vi "setTics.vi"(6 "AdditionalTics":dbl[](array[numeric]), 7 "tics":T3={"ticMin"=0.0, "ticStep"=0.0, "ticMax"=0.0, "minorDivsPerMajor"=2, "ticSpacing"=enum."Auto Tics", "ticPosition"=enum."Inside, no mirror"}, 8 "AxisSpan":dbl, 9 "Axis":T2, 11 "String in":string) -> (0 "polarGrid":dbl, 3 "String out":string)   [LabVIEW 2013]
uses:
  tics.ctl
  axisName.ctl
  commandArray.ctl
panel:
  out "Commands":T1
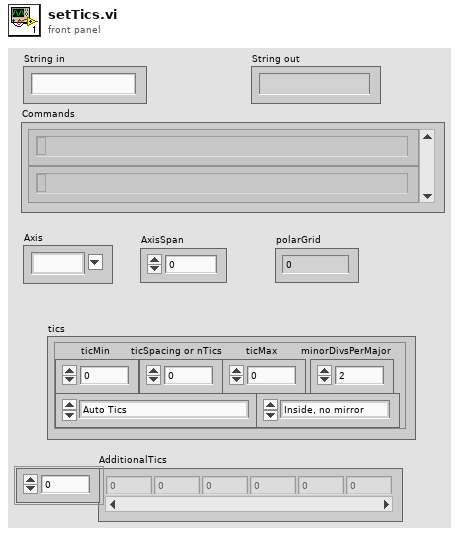
[diagram p1: front panel]
types:
  T1 = typedef "commandArray.ctl" = string[]
  T2 = typedef "axisName.ctl" = string
  T3 = typedef "tics.ctl" = cluster{"ticMin":dbl, "ticStep":dbl, "ticMax":dbl, "minorDivsPerMajor":i32, "ticSpacing":enum16{"Auto Tics", "Fixed spacing", "Fixed Minimum and Spacing", "Start, Spacing and Maximum", "Approx n Tics (rounded)"}, "ticPosition":enum16{"Inside, no mirror", "Inside, mirrored", "Outside, no mirror", "Outside, mirrored", "Invisible"}}
  T4 = enum16{"Auto Tics", "Fixed spacing", "Fixed Minimum and Spacing", "Start, Spacing and Maximum", "Approx n Tics (rounded)"}
  T5 = enum16{"Inside, no mirror", "Inside, mirrored", "Outside, no mirror", "Outside, mirrored", "Invisible"}
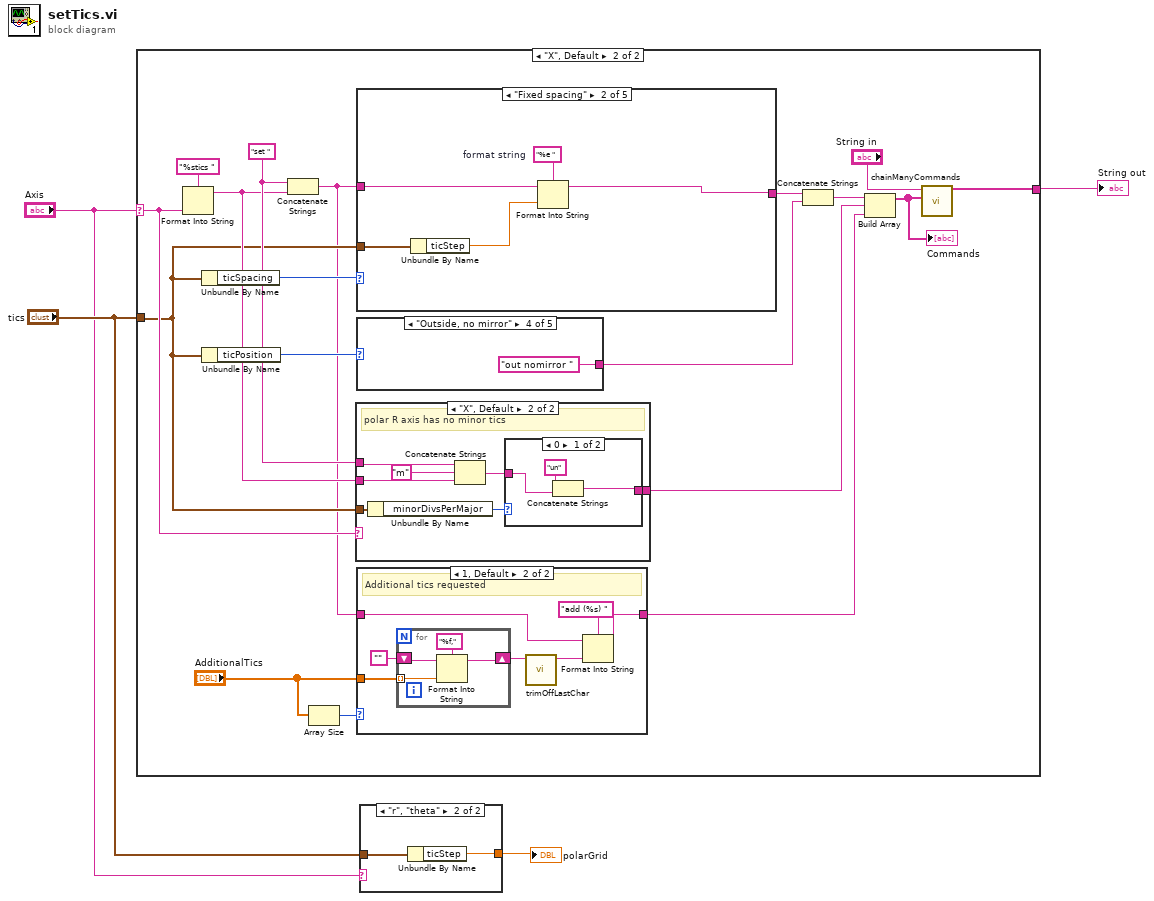
[diagram p0: block diagram]
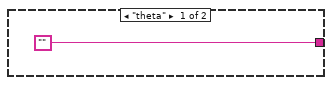
[diagram p2: hidden frame]
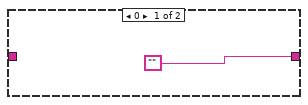
[diagram p3: hidden frame]
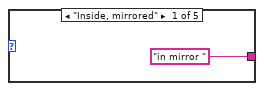
[diagram p4: hidden frame]
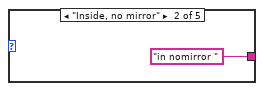
[diagram p5: hidden frame]
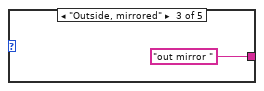
[diagram p6: hidden frame]
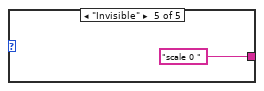
[diagram p7: hidden frame]
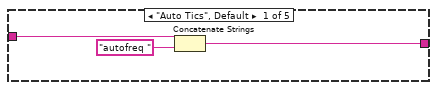
[diagram p8: hidden frame]
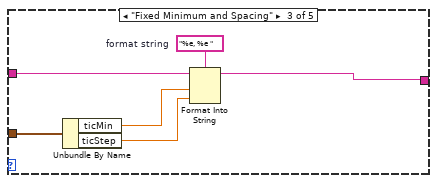
[diagram p9: hidden frame]
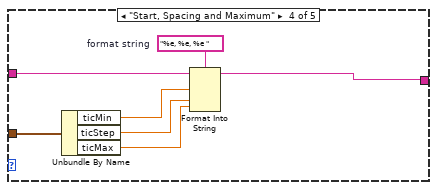
[diagram p10: hidden frame]
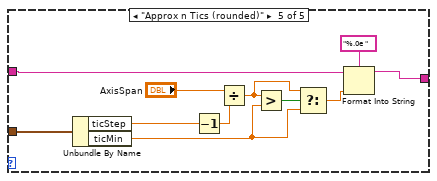
[diagram p11: hidden frame]
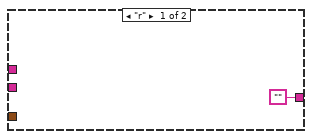
[diagram p12: hidden frame]
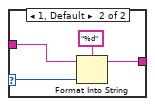
[diagram p13: hidden frame]
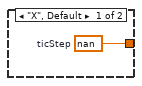
[diagram p14: hidden frame]
diagram:
  n1 = case shown="\"X\", Default" "Axis" {
    selector: "Axis" -> [_ w17]
    tunnel: ["" w22] -> w4
    tunnel: "tics" -> [_ w13]
    frame "theta" {
    }
    frame "X", Default {
      w16 = "set " ("format string")
      n2 = Format Into String(format string="%stics ", w17) -> (resulting string=w15:string)  [unwired: 2 in, 1 out]
      n3 = Unbundle By Name(w13) -> ("ticSpacing"=w12:T4)
      n4 = Unbundle By Name(w13) -> ("ticPosition"=w11:T5)
      n5 = Concatenate Strings(w16, w15) -> (w7:string)
      n6 = Array Size(array="AdditionalTics") -> (size(s)=w9:i32)
      n7 = case shown="\"X\", Default" w17 {
        tunnel: w16 -> [_ w79]
        tunnel: w15 -> [_ w78]
        tunnel: ["" w75] -> w19
        tunnel: w13 -> [_ w74]
        frame "r" {
        }
        frame "X", Default {
          # "polar R axis has no minor tics"
          n8 = Unbundle By Name(w74) -> ("minorDivsPerMajor"=w80:i32)
          n9 = Concatenate Strings(w79, "m" ("string"), w78) -> (w76:string)
          n10 = case shown="0" w80 {
            selector: w80 -> [_ w85]
            tunnel: w76 -> [w83 w86]
            tunnel: [w82 w84] -> w75
            frame 0 {
              n11 = Concatenate Strings("un" ("string"), w83) -> (w82:string)
            }
            frame 1, Default {
              n12 = Format Into String(format string="%d", initial string=w86, w85) -> (resulting string=w84:string)  [unwired: 1 in, 1 out]
            }
          }
        }
      }
      n13 = case shown="\"Fixed spacing\"" w12 {
        tunnel: w7 -> [w43 w48 w54 w61 w62]
        tunnel: [w42 w44 w50 w57 w72] -> w14
        tunnel: w13 -> [_ w47 w53 w60 w71]
        frame "Auto Tics", Default {
          n14 = Concatenate Strings(w43, "autofreq " ("string")) -> (w42:string)
        }
        frame "Fixed spacing" {
          w45 = "%e "  # format string
          n15 = Unbundle By Name(w47) -> ("ticStep"=w46:dbl)
          n16 = Format Into String(format string=w45, initial string=w48, w46) -> (resulting string=w44:string)  [unwired: 1 in, 1 out]
        }
        frame "Fixed Minimum and Spacing" {
          w51 = "%e, %e "  # format string
          n17 = Unbundle By Name(w53) -> ("ticMin"=w52:dbl, "ticStep"=w49:dbl)
          n18 = Format Into String(format string=w51, initial string=w54, w52, w49) -> (resulting string=w50:string)  [unwired: 1 in, 1 out]
        }
        frame "Start, Spacing and Maximum" {
          w58 = "%e, %e, %e "  # format string
          n19 = Unbundle By Name(w60) -> ("ticMin"=w59:dbl, "ticStep"=w56:dbl, "ticMax"=w55:dbl)
          n20 = Format Into String(format string=w58, initial string=w61, w59, w56, w55) -> (resulting string=w57:string)  [unwired: 1 in, 1 out]
        }
        frame "Approx n Tics (rounded)" {
          n21 = Unbundle By Name(w71) -> ("ticStep"=w64:dbl, "ticMin"=w65:dbl)
          n22 = Decrement(x=w64) -> (x-1=w66:dbl)
          n23 = Divide(x="AxisSpan", y=w66) -> (x/y=w69:dbl)
          n24 = Greater?(x=w69, y=w65) -> (0:w68:bool)
          n25 = Select(t=w69, s=w68, f=w65) -> (s? t:f=w70:dbl)
          n26 = Format Into String(format string="%.0e ", initial string=w62, w70) -> (resulting string=w72:string)  [unwired: 1 in, 1 out]
        }
      }
      n27 = case shown="\"Outside, no mirror\"" w11 {
        tunnel: ["in mirror " "in nomirror " "out mirror " "out nomirror " "scale 0 "] -> w10
        frame "Inside, mirrored" {
        }
        frame "Inside, no mirror" {
        }
        frame "Outside, mirrored" {
        }
        frame "Outside, no mirror" {
        }
        frame "Invisible" {
        }
      }
      n28 = case shown="1, Default" w9 {
        tunnel: ["" w30] -> w8
        tunnel: w7 -> [_ w31]
        tunnel: "AdditionalTics" -> [_ w28]
        frame 0 {
        }
        frame 1, Default {
          # "Additional tics requested"
          n29 = for {
            tunnel: w28 -> [w35] mode=indexing
            shift-right: [w32] -> w26
            shift-left: "" -> [w33]
            n30 = Format Into String(format string="%f,", initial string=w33, w35) -> (resulting string=w32:string)  [unwired: 1 in, 1 out]
          }
          n31 = call "trimOffLastChar.vi"("String in"=w26) -> ("String out"=w25:string)  [unwired: 10 in]
          n32 = Format Into String(format string="add (%s) ", initial string=w31, w25) -> (resulting string=w30:string)  [unwired: 1 in, 1 out]
        }
      }
      n33 = Concatenate Strings(w14, w10) -> (w20:string)
      n34 = Build Array(w20, w19, w8) -> (w18:string[])
      "Commands" <- w18
      n35 = call "chainManyCommands.vi"("CommandArray"=w18, "String in in"="String in") -> ("String out"=w22:string)  [unwired: 9 in]
    }
  }
  "String out" <- w4
  n36 = case shown="\"r\", \"theta\"" "Axis" {
    tunnel: "tics" -> [_ w90]
    tunnel: [w88 w89] -> w2
    frame "X", Default {
      w88 = nan  # ticStep
    }
    frame "r", "theta" {
      n37 = Unbundle By Name(w90) -> ("ticStep"=w89:dbl)
    }
  }
  "polarGrid" <- w2
